vi "Parse Response JSON.vi"(8 "error in (no error)":errorcluster, 10 "Response JSON":string, 11 "RGetInputVolume in":refnum<class "RGetInputVolume.lvclass">) -> (0 "error out":errorcluster, 3 "RGetInputVolume out":refnum<class "RGetInputVolume.lvclass">)   [LabVIEW 2020, in "obs-websocket.lvlib" / "RGetInputVolume.lvclass"]
uses:
  RGetInputVolume.lvclass
  RGetInputVolume.lvclass/RGetInputVolume.ctl
  2b2c4f29-094a-4369-99a2-01466997c2a4.vi
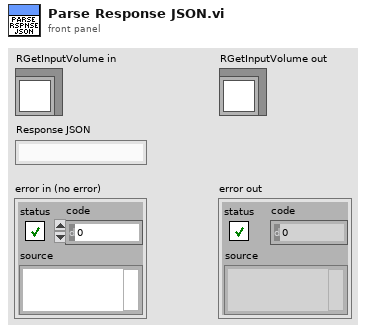
[diagram p1: front panel]
types:
  T1 = cluster{"inputVolumeMul":dbl, "inputVolumeDb":dbl}
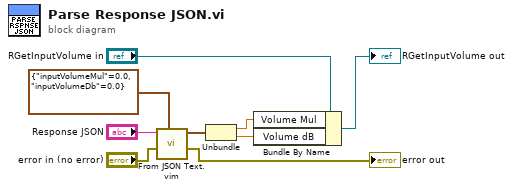
[diagram p0: block diagram]
diagram:
  n1 = call "From JSON Text.vim"("Data Type and Default Value"=T1 {"inputVolumeMul"=0.0, "inputVolumeDb"=0.0}, "error in (no error)"="error in (no error)", "JSON"="Response JSON") -> ("error out"=→"error out":errorcluster, "Data out"=w3:T1)  [unwired: 7 in]
  n2 = Unbundle(w3) -> ("inputVolumeMul"=w2:dbl, "inputVolumeDb"=w1:dbl)
  n3 = Bundle By Name(cluster="RGetInputVolume in", "Volume Mul"=w2, "Volume dB"=w1) -> (→"RGetInputVolume out":refnum<class "RGetInputVolume.lvclass">)
